vi "Construct Json Data Reader.vi"(5 "Json Data Reader in":refnum<class "Json Data Reader.lvclass">, 8 "error in (no error)":errorcluster, 11 "Json File":path) -> (0 "error out":errorcluster, 3 "Json Data Reader":refnum<class "Json Data Reader.lvclass">)   [LabVIEW 2017, in "Json Data Reader.lvclass"]
uses:
  Json Data Reader.lvclass
  Json Data Reader.lvclass/Json Data Reader.ctl
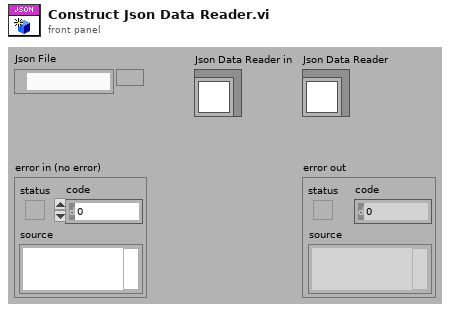
[diagram p1: front panel]
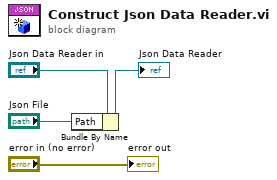
[diagram p0: block diagram]
diagram:
  n1 = Bundle By Name(cluster="Json Data Reader in", "Path"="Json File") -> (→"Json Data Reader":refnum<class "Json Data Reader.lvclass">)
  "error out" <- "error in (no error)"
